vi "4 Bits Initialize Entry.vi"(6 "E?E1:E2 (E1)":bool=TRUE, 11 "device connection map":T1={"RS"="RS", "R/W"="RW", "E1"="E1", "E2"="E2", "DB4"="DB4", "DB5"="DB5", "DB6"="DB6", "DB7"="DB7"}) -> ()   [LabVIEW 2017, in "HD44780 FPGA.lvlib"]
uses:
  HD44780 FPGA.lvlib
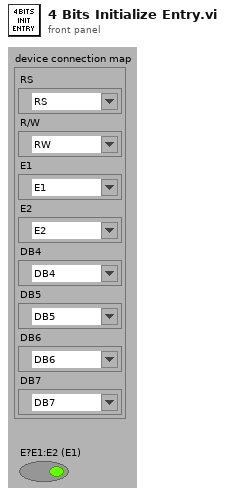
[diagram p1: front panel]
types:
  T1 = cluster{"RS":refnum<k21>, "R/W":refnum<k21>, "E1":refnum<k21>, "E2":refnum<k21>, "DB4":refnum<k21>, "DB5":refnum<k21>, "DB6":refnum<k21>, "DB7":refnum<k21>}
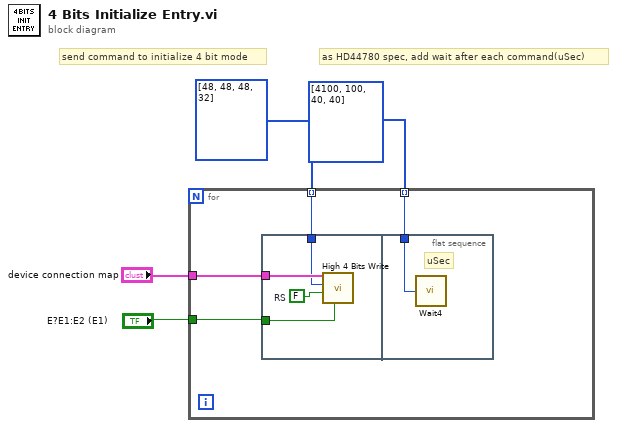
[diagram p0: block diagram]
diagram:
  # "send command to initialize 4 bit mode"
  # "as HD44780 spec, add wait after each command(uSec)"
  n1 = for {
    tunnel: "device connection map" -> [w8]
    tunnel: "E?E1:E2 (E1)" -> [w7]
    tunnel: u8[] [48, 48, 48, 32] ("initialized array") -> [w6] mode=indexing
    tunnel: u16[] [4100, 100, 40, 40] ("initialized array") -> [w5] mode=indexing
    n2 = flat-sequence {
      tunnel: w8 -> [w12]
      tunnel: w7 -> [w10]
      tunnel: w6 -> [w9]
      tunnel: w5 -> [w13]
      frame #0 {
        w11 = FALSE  # RS
        n3 = call "High 4 Bits Write.vi"("E?E1:E2 (E1)"=w10, "RS"=w11, "LCD data/cmd"=w9, "device connection map"=w12) -> ()  [unwired: 8 in]
      }
      frame #1 {
        # "uSec"
        n4 = call "Wait4"("Count(uSec)"=w13) -> ()  [unwired: 1 out]
      }
    }
  }
